vi "Serialize a JSON Serializable Object.vi"() -> ()   [LabVIEW 2017]
doc: "Demonstrates the JSONtext Object Serializer by serializing a LabVIEW Object - that inherits from JSON Serializable - to JSON."
uses:
  JSON Serializable Serializer/JSON Serializable Serializer.lvclass
  C:/Program Files (x86)/National Instruments/LabVIEW 2017/vi.lib/JDP Science/JSONtext/LVClass Serializer/JSONtext LVClass Serializer.lvclass
  585c77a6-94ca-412b-a7e9-3a1ed3474501.vi
  <vilib>/JDP Science/JSONtext/Variant to JSON Text.vi
  Serializable Account/Serializable Account.lvclass
panel:
  in  "CreatedDate":timestamp=timestamp(3700276200 s since 1904-01-01)
  in  "Active":bool=TRUE
  in  "Email":string="john.doe@example.com"
  in  "Roles":string[](array[string])=["User", "Admin"]
  out "error out":errorcluster
  out "<JSON>":string
  # "Overview\nDemonstrates the JSONtext Object Serializer by serializing a LabVIEW Object - that inherits from JSON Serializable - to JSON.\n\nInstructions\nRun the VI"
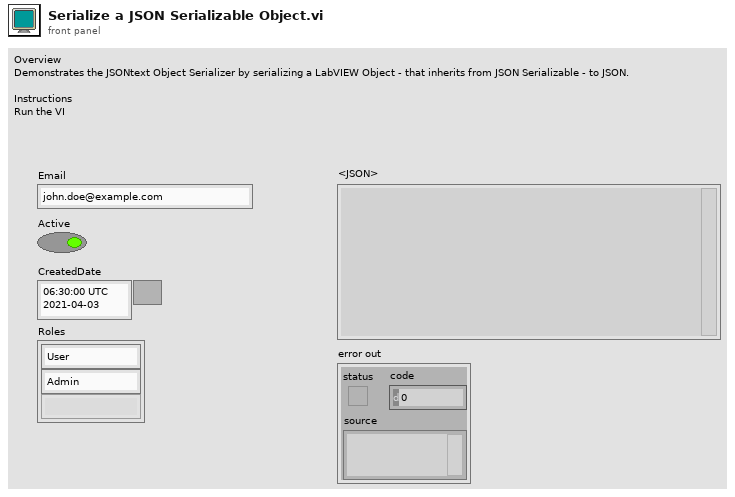
[diagram p1: front panel]
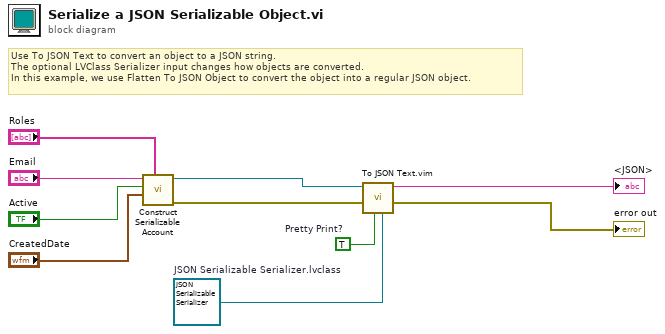
[diagram p0: block diagram]
diagram:
  w4 = refnum<class "JSON Serializable Serializer.lvclass"> refnum  # JSON Serializable Serializer.lvclass
  w5 = TRUE  # Pretty Print?
  # "Use To JSON Text to convert an object to a JSON string.\nThe optional LVClass Serializer input changes how objects are converted.\nIn this example, we use Flatten To JSON Object to convert the object into a regular JSON object."
  n1 = call "Construct Serializable Account.vi"("Roles"="Roles", "CreatedDate"="CreatedDate", "Active"="Active", "Email"="Email") -> ("error out"=w6:errorcluster, "Serializable Account"=w1:refnum<class "Serializable Account.lvclass">)  [unwired: 6 in]
  n2 = call "To JSON Text.vim"("LVClass Serializer"=w4, "Pretty Print?"=w5, "error in (no error)"=w6, "Anything"=w1) -> ("error out"=→"error out":errorcluster, "<JSON>"=→"<JSON>":string)  [unwired: 6 in]
